vi "Configure Trigger.vi"(8 "error in (no error)":errorcluster, 11 "DAQmx Base CFG in":refnum<class "DAQmx Base CFG.lvclass">) -> (0 "error out":errorcluster, 3 "DAQmx Base CFG out":refnum<class "DAQmx Base CFG.lvclass">)   [LabVIEW 2023, in "DAQmx Base CFG.lvclass"]
uses:
  DAQmx Base CFG.lvclass
  D:/git/HAL/HAL GOOP4/Configuration JSON Base/CFG JSON Base.lvclass
  Configuration JSON Base/CFG JSON Base.lvclass/CFG JSON Base.ctl
  bd3d4a76-19b6-4dfd-953c-4f45e38a3d65.vi
  <vilib>/JDP Science/JSONtext/Find Item.vi
  <vilib>/JDP Science/JSONtext/Next JSON Value.vi
  <vilib>/JDP Science/JSONtext/String Subset.vi
  <vilib>/JDP Science/JSONtext/Parsing/Advance past next JSON Value (inlined COPY).vi
  <vilib>/JDP Science/JSONtext/Parsing/Advance past whitespace.vi
  <vilib>/JDP Science/JSONtext/Parsing/Advance past String.vi
  <vilib>/JDP Science/JSONtext/Parsing/Advance past Number.vi
  <vilib>/JDP Science/JSONtext/Parsing/Advance past Line Ending.vi
  <vilib>/JDP Science/JSONtext/Parsing/Parse Full Path or Item Name.vi
  <vilib>/JDP Science/JSONtext/Parsing/Advance past Array.vi
  <vilib>/JDP Science/JSONtext/Parsing/Advance past Object.vi
  <vilib>/JDP Science/JSONtext/support/Error Cluster From Code.vi
  <vilib>/JDP Science/JSONtext/Offset/Find Item Locations by Path.vi
  <vilib>/JDP Science/JSONtext/JSON text to Variant.vi
  <vilib>/Utility/error.llb/Error Cluster From Error Code.vi
  <vilib>/JDP Science/JSONtext/LVClass Serializer/JSONtext LVClass Serializer.lvclass
  <vilib>/ErrorRing/Error Ring.xnode
  Configuration JSON Base/CFG JSON Base.lvclass
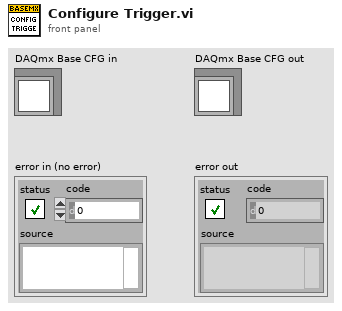
[diagram p1: front panel]
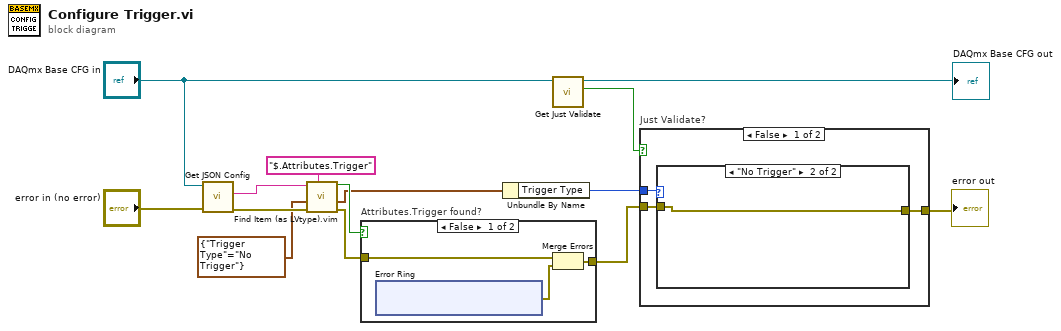
[diagram p0: block diagram]
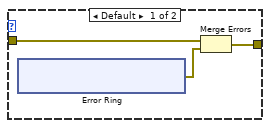
[diagram p2: hidden frame]
diagram:
  n1 = call "Get JSON Config.vi"("error in (no error)"="error in (no error)", "CFG Base in"="DAQmx Base CFG in") -> ("error out"=w14:errorcluster, "<JSON>Config>"=w13:string)  [unwired: 7 in, 1 out]
  n2 = call "Find Item (as LVtype).vim"("$Path or Item Name"="$.Attributes.Trigger", "error in (no error)"=w14, "Data Type and Default Value"=cluster{"Trigger Type":enum16{"No Trigger"}} {"Trigger Type"=enum."No Trigger"}, "JSON"=w13) -> ("error out"=w10:errorcluster, "Data"=w8:cluster{"Trigger Type":enum16{"No Trigger"}}, "Found"=w9:bool)  [unwired: 4 in, 1 out]
  n3 = case "Attributes.Trigger found?" shown="False" w9 {
    tunnel: w10 -> [w16 w23]
    tunnel: [w15 w23] -> w6
    frame False {
      n4 = xnode "Error Ring"() -> ("error out"=w17:errorcluster)
      n5 = Merge Errors(w16, w17) -> (w15:errorcluster)
    }
    frame True {
    }
  }
  n6 = Unbundle By Name(w8) -> ("Trigger Type"=w7:enum16{"No Trigger"})
  n7 = call "Get Just Validate.vi"("CFG JSON Base in"="DAQmx Base CFG in") -> ("Just Validate"=w1:bool, "CFG JSON Base out"=→"DAQmx Base CFG out":refnum<class "DAQmx Base CFG.lvclass">)  [unwired: 8 in, 1 out]
  n8 = case "Just Validate?" shown="False" w1 {
    tunnel: w7 -> [w26 _]
    tunnel: w6 -> [w25 w36]
    tunnel: [w24 w36] -> w4
    frame False {
      n9 = case shown="\"No Trigger\"" w26 {
        tunnel: w25 -> [w29 w35]
        tunnel: [w27 w35] -> w24
        frame Default {
          n10 = xnode "Error Ring"() -> ("error out"=w28:errorcluster)
          n11 = Merge Errors(w29, w28) -> (w27:errorcluster)
        }
        frame "No Trigger" {
        }
      }
    }
    frame True {
    }
  }
  "error out" <- w4
